vi "Main.vi"(8 "error in":errorcluster, 11 "About View in":refnum<class "About View.lvclass">) -> (0 "error out":errorcluster, 3 "About View out":refnum<class "About View.lvclass">)   [LabVIEW 2018, in "About View.lvclass"]
doc: "The Queued Message Handler of a Worker."
uses:
  About View.lvclass
  Initialization Data.ctl
  About View.lvclass/About View.ctl
panel:
  # "I  hope  that  Workers?  will  be  able  to  increase  the  productivity  of  novice  and  advanced \ndevelopers alike, allowing you to develop larger projects in less time, and with less complexity."
  # "Workers Demo -- Aging Test"
  # "designed by Retry, 2022"
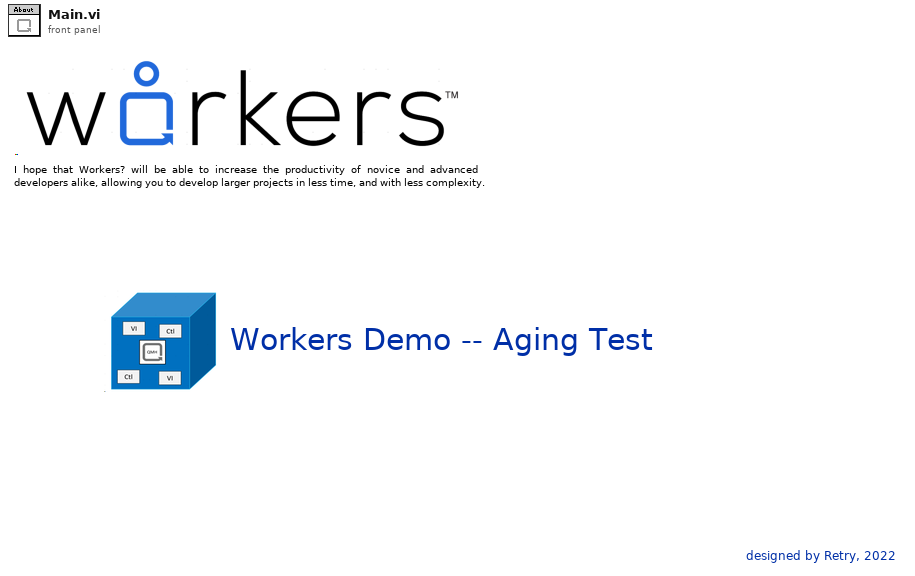
[diagram p1: front panel]
types:
  T1 = typedef "About View.lvclass/Initialization Data.ctl" = cluster{"MainPanel":refnum<vi>}
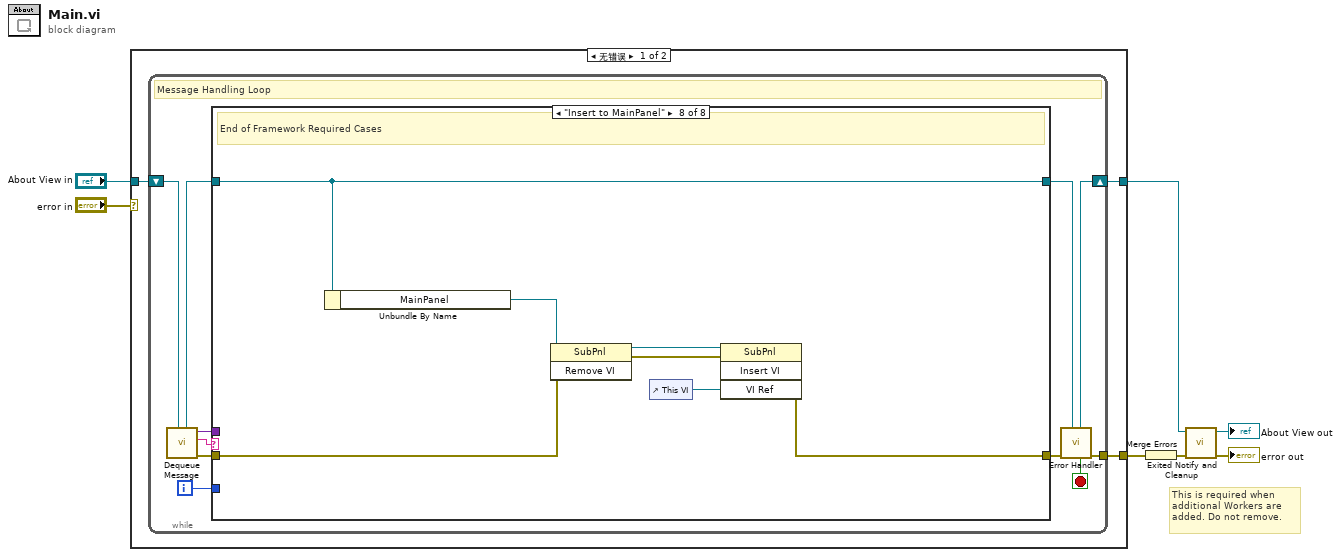
[diagram p0: block diagram]
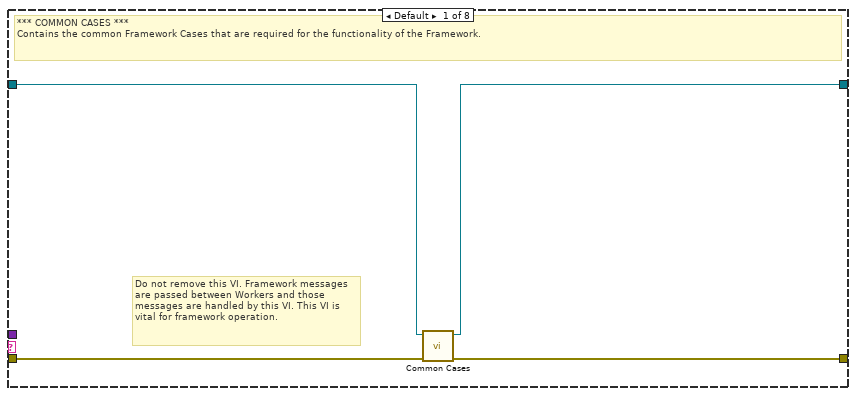
[diagram p2: hidden frame]
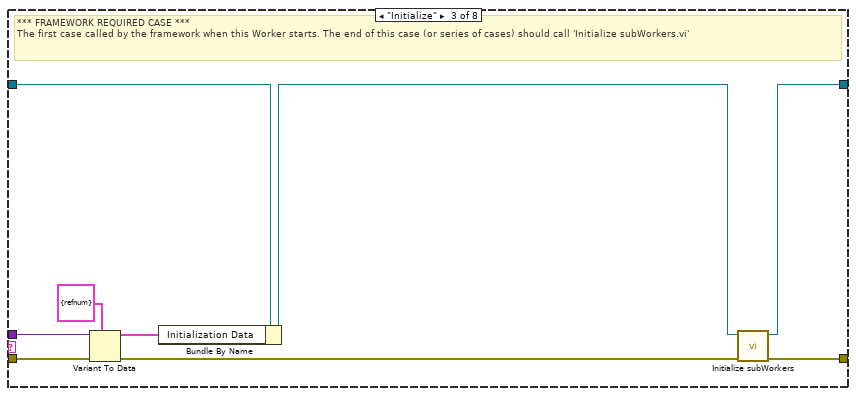
[diagram p4: hidden frame]
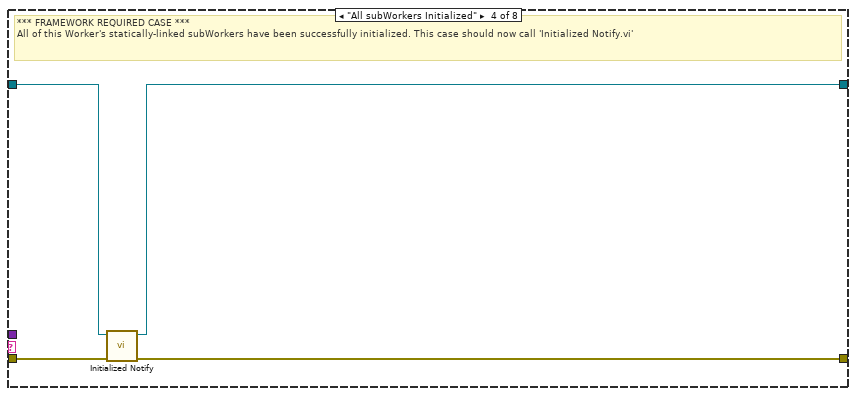
[diagram p5: hidden frame]
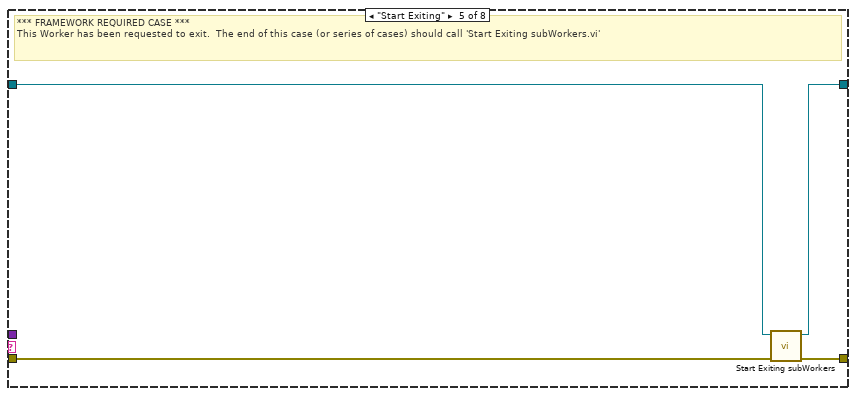
[diagram p6: hidden frame]
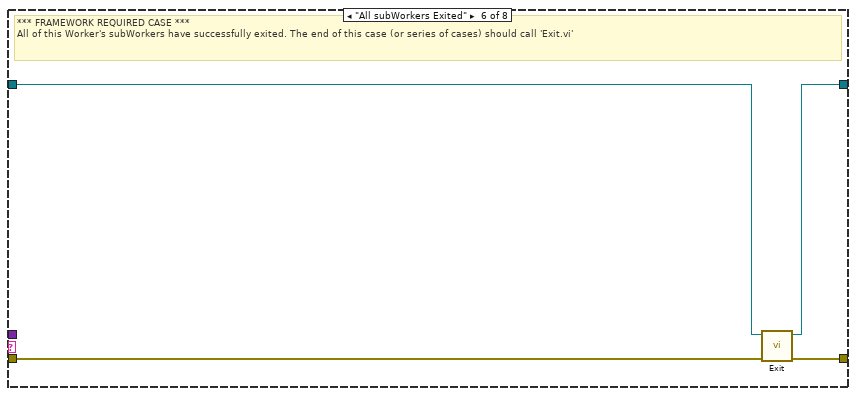
[diagram p7: hidden frame]
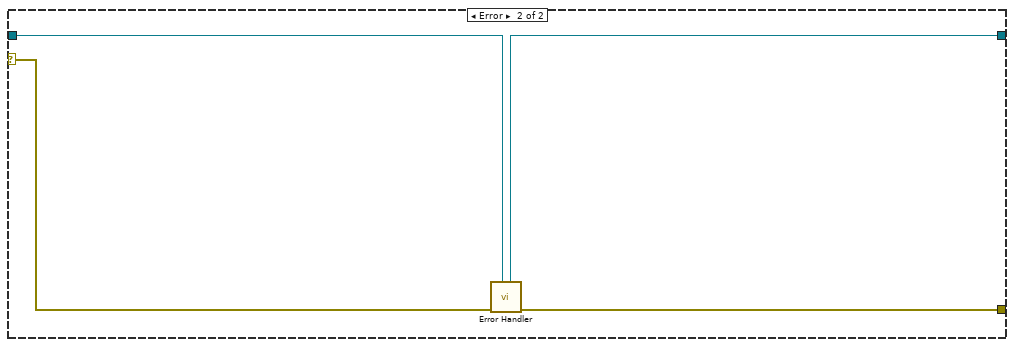
[diagram p9: hidden frame]
diagram:
  # "This is required when additional Workers are added. Do not remove."
  n1 = case shown="无错误" "error in" {
    tunnel: "About View in" -> [w8 w59]
    tunnel: [w10 w60] -> w6
    tunnel: [w9 w58] -> w7
    selector: "error in" -> [_ w61]
    frame No Error {
      n2 = while {
        shift-right: [w19] -> w9
        shift-left: w8 -> [w21]
        tunnel: [w20] -> w10
        i -> [w11]
        stop <- w12 stop-if-true
        # "Message Handling Loop"
        n3 = call-dynamic "Dequeue Message.vi"("Worker"=w21) -> ("error out"=w18:errorcluster, "Case out"=w13:string, "Data out"=w14:variant, "Worker out"=w16:refnum<class "About View.lvclass">)  [unwired: 6 in, 1 out]
        n4 = case "Worker MHL Case Structure (DO NOT CHANGE LABEL NAME)" shown="\"Insert to MainPanel\"" w13 {
          tunnel: w18 -> [w25 w26 w34 w40 w41 w48 w49 w52]
          tunnel: [w24 w26 w36 w39 w44 w47 w49 w51] -> w17
          tunnel: w16 -> [w23 w27 w33 w38 w42 w46 w50 w53]
          tunnel: [w22 w27 w35 w37 w43 w45 w50 w53] -> w15
          tunnel: w14 -> [_ _ w31 _ _ _ _ _]
          tunnel: w11 -> [_ _ _ _ _ _ _ _]
          frame Default {
            # "Do not remove this VI. Framework messages are passed between Workers and those messages are handled by this VI. This VI is vital for framework operation."
            # "*** COMMON CASES ***\nContains the common Framework Cases that are required for the functionality of the Framework."
            n5 = call-dynamic "Common Cases.vi"("error in"=w25, "Worker in"=w23) -> ("error out"=w24:errorcluster, "Worker out"=w22:refnum<class "About View.lvclass">)  [unwired: 8 in]
          }
          frame "------ FRAMEWORK REQUIRED CASES ------" {
            # "Start of Framework Required Cases"
          }
          frame "Initialize" {
            # "*** FRAMEWORK REQUIRED CASE ***\nThe first case called by the framework when this Worker starts. The end of this case (or series of cases) should call 'Initialize subWorkers.vi'"
            n6 = Variant To Data(error in=w34, type=T1 {"MainPanel"=refnum} ("Cluster"), Variant=w31) -> (data=w28:T1, error out=w32:errorcluster)
            n7 = Bundle By Name(cluster=w33, "Initialization Data"=w28) -> (w30:refnum<class "About View.lvclass">)
            n8 = call-dynamic "Initialize subWorkers.vi"("error in"=w32, "Worker"=w30) -> ("error out"=w36:errorcluster, "dup Worker out"=w35:refnum<class "About View.lvclass">)  [unwired: 8 in]
          }
          frame "All subWorkers Initialized" {
            # "*** FRAMEWORK REQUIRED CASE ***\nAll of this Worker's statically-linked subWorkers have been successfully initialized. This case should now call 'Initialized Notify.vi'"
            n9 = call-dynamic "Initialized Notify.vi"("error in"=w40, "Worker"=w38) -> ("error out"=w39:errorcluster, "dup Worker out"=w37:refnum<class "About View.lvclass">)  [unwired: 8 in]
          }
          frame "Start Exiting" {
            # "*** FRAMEWORK REQUIRED CASE ***\nThis Worker has been requested to exit.  The end of this case (or series of cases) should call 'Start Exiting subWorkers.vi'"
            n10 = call-dynamic "Start Exiting subWorkers.vi"("error_in"=w41, "Worker"=w42) -> ("error out"=w44:errorcluster, "dup Worker out"=w43:refnum<class "About View.lvclass">)  [unwired: 8 in]
          }
          frame "All subWorkers Exited" {
            # "*** FRAMEWORK REQUIRED CASE ***\nAll of this Worker's subWorkers have successfully exited. The end of this case (or series of cases) should call 'Exit.vi'"
            n11 = call-dynamic "Exit.vi"("error_in"=w48, "Worker"=w46) -> ("error out"=w47:errorcluster, "dup Worker out"=w45:refnum<class "About View.lvclass">)  [unwired: 8 in]
          }
          frame "-----------------------------------------------" {
            # "End of Framework Required Cases"
          }
          frame "Insert to MainPanel" {
            # "End of Framework Required Cases"
            n12 = Unbundle By Name(w53) -> ("MainPanel"=w57:refnum<vi>)
            n13 = invoke class="SubPnl" method="Remove VI"(reference=w57, error in=w52) -> (reference out=w56:refnum<vi>, error out=w55:errorcluster)  [unwired: 1 in, 1 out]
            n14 = control-ref of="This VI"() -> (w54:refnum<vi>)
            n15 = invoke class="SubPnl" method="Insert VI"(reference=w56, error in=w55, "VI Ref"=w54) -> (error out=w51:errorcluster)  [unwired: 1 in, 3 out]
          }
        }
        n16 = call-dynamic "Error Handler.vi"("Worker"=w15, "error_in"=w17) -> ("error out"=w20:errorcluster, "Stop Loop"=w12:bool, "Worker out"=w19:refnum<class "About View.lvclass">)  [unwired: 7 in]
      }
    }
    frame Error {
      n17 = call-dynamic "Error Handler.vi"("Worker"=w59, "error_in"=w61) -> ("error out"=w60:errorcluster, "Worker out"=w58:refnum<class "About View.lvclass">)  [unwired: 7 in, 1 out]
    }
  }
  n18 = Merge Errors(w6) -> (w3:errorcluster)
  n19 = call-dynamic "Exited Notify and Cleanup.vi"("error_in"=w3, "Worker"=w7) -> ("error out"=→"error out":errorcluster, "dup Worker out"=→"About View out":refnum<class "About View.lvclass">)  [unwired: 8 in]
